vi "VI Get Mods.vi"(8 "error in (no error)":errorcluster, 11 "vi reference":refnum<vi>) -> (0 "error out":errorcluster, 2 "Modified?":bool, 3 "dup vi reference":refnum<vi>)   [LabVIEW 2009]
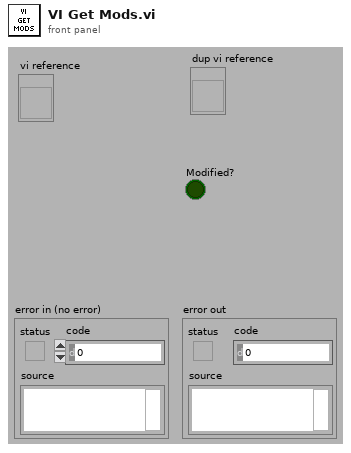
[diagram p1: front panel]
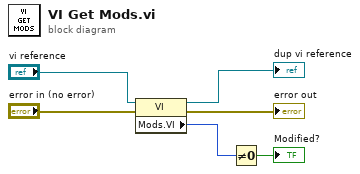
[diagram p0: block diagram]
diagram:
  n1 = property class="VI"(reference="vi reference", error in="error in (no error)") -> (reference out=→"dup vi reference":refnum<vi>, error out=→"error out":errorcluster, "Mods.VI"=w5:u64)
  n2 = Not Equal To 0?(x=w5) -> (x != 0?=→"Modified?":bool)
